vi "Client Download Tests and Drivers.vi"(8 "error in (no error)":errorcluster, 9 "Test or Driver URL Path (empty)":path, 10 "ServerPort (80)":u16=80, 11 "Server (\"\")":string) -> (0 "error out":errorcluster)   [LabVIEW 2011]
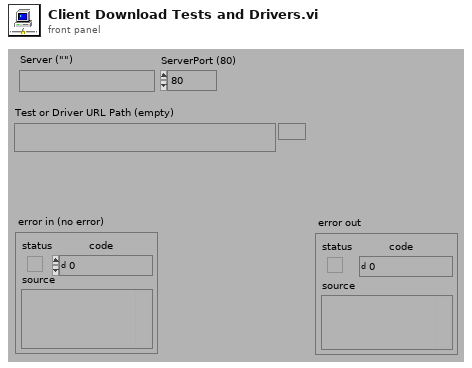
[diagram p1: front panel]
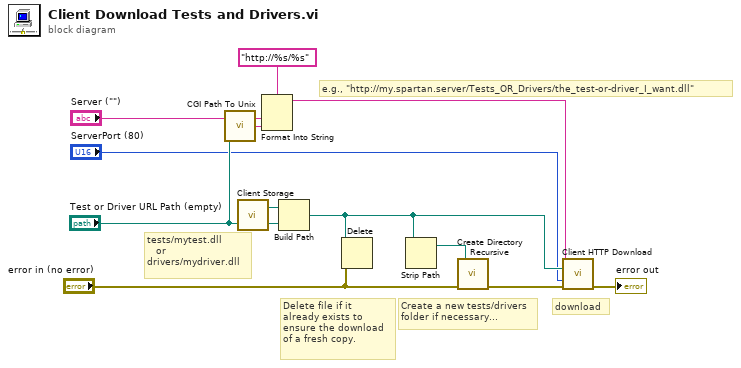
[diagram p0: block diagram]
diagram:
  # "Delete file if it\nalready exists to\nensure the download\nof a fresh copy."
  # "download"
  # "Create a new tests/drivers\nfolder if necessary..."
  # "tests/mytest.dll\n   or\ndrivers/mydriver.dll"
  # "e.g., \"http://my.spartan.server/Tests_OR_Drivers/the_test-or-driver_I_want.dll\""
  n1 = call "CGI Path To Unix.vi"("platform path"="Test or Driver URL Path (empty)") -> ("unix path"=w2:string)  [unwired: 1 in]
  n2 = call "Client Storage.vi"() -> ("Client Storage Path"=w9:path)  [unwired: 3 in]
  n3 = Format Into String(format string="http://%s/%s" ("name (unnamed)"), "Server (\"\")", w2) -> (resulting string=w4:string)  [unwired: 2 in, 1 out]
  n4 = Build Path(base path=w9, name or relative path="Test or Driver URL Path (empty)") -> (appended path=w7:path)
  n5 = Delete(path (use dialog)=w7, error in="error in (no error)") -> ()  [unwired: 6 out]
  n6 = Strip Path(path=w7) -> (stripped path=w8:path)  [unwired: 1 out]
  n7 = call <vilib>:"Create Directory Recursive.vi"("error in (no error)"="error in (no error)", "directory"=w8) -> ("error out"=w10:errorcluster)  [unwired: 1 in, 4 out]
  n8 = call "Client HTTP Download.vi"("http URL"=w4, "file path (Not A Path)"=w7, "Port (80)"="ServerPort (80)", "error in (no error)"=w10) -> ("error out"=→"error out":errorcluster)  [unwired: 1 in, 10 out]
